vi "b2.vi"   [LabVIEW 2020]
uses:
  <instrlib>/Agilent B2900 Series/Agilent B2900 Series.lvlib
  <instrlib>/Agilent B2900 Series/Public/Data/Low Level/Fetch Measurement (Multiple Points).vi
  <instrlib>/Agilent B2900 Series/Public/Configure/Measurement/Configure Measurement (Resistance).vi
  <instrlib>/Agilent B2900 Series/Public/Data/Read Measurement Result (Single Point).vi
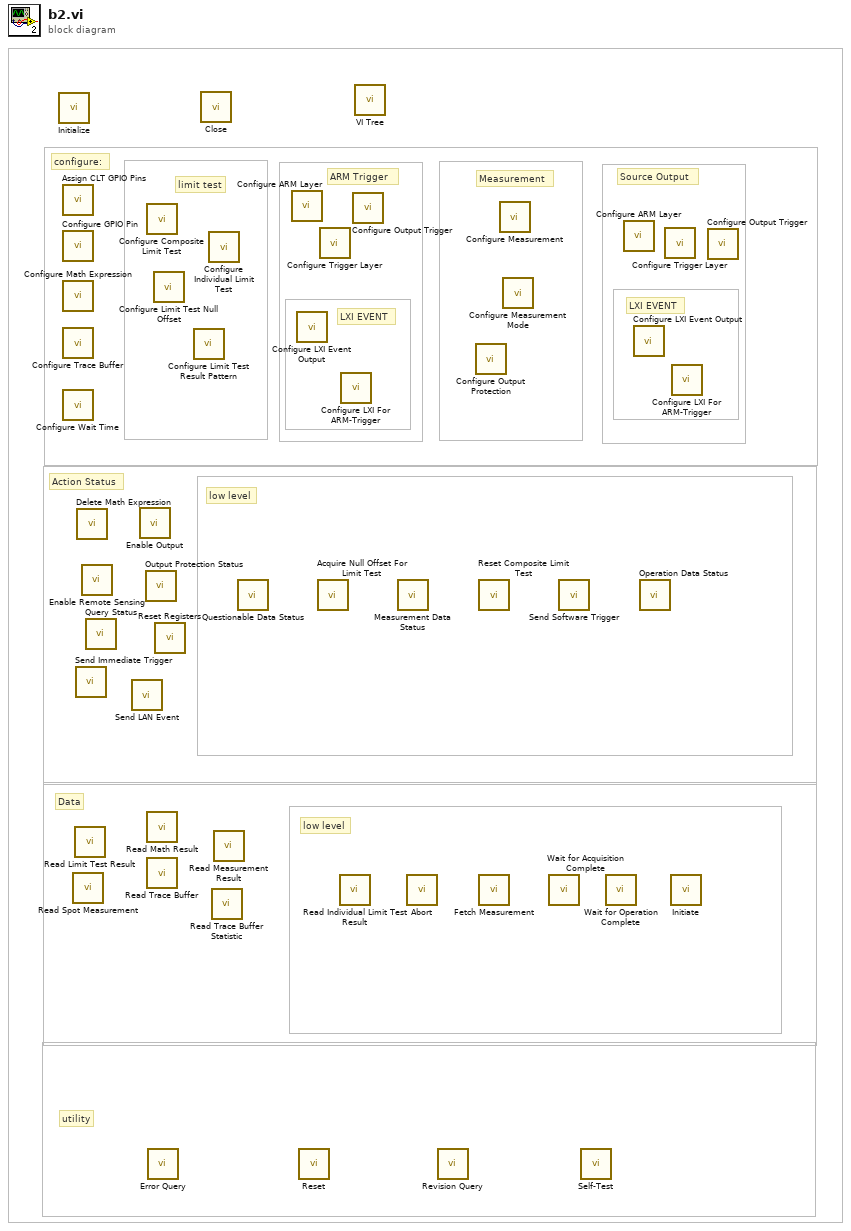
[diagram p0: block diagram]
diagram:
  # "utility"
  # "low level"
  # "low level"
  # "Data"
  # "Action Status"
  # "Source Output"
  # "Measurement"
  # "LXI EVENT"
  # "LXI EVENT"
  # "ARM Trigger"
  # "limit test"
  # "configure:"
  n1 = call <instrlib>:"Initialize.vi"() -> ()  [unwired: 10 in, 2 out]
  n2 = call <instrlib>:"Assign CLT GPIO Pins.vi"() -> ()  [unwired: 10 in, 2 out]
  n3 = call <instrlib>:"Configure GPIO Pin.vi"() -> ()  [unwired: 14 in, 2 out]
  n4 = call <instrlib>:"Configure Math Expression.vi"() -> ()  [unwired: 10 in, 2 out]
  n5 = call <instrlib>:"Configure Trace Buffer.vi"() -> ()  [unwired: 10 in, 2 out]
  n6 = call <instrlib>:"Configure Wait Time.vi"() -> ()  [unwired: 14 in, 2 out]
  n7 = call <instrlib>:"Read Spot Measurement.vi"() -> ()  [unwired: 9 in, 3 out]
  n8 = call <instrlib>:"Read Limit Test Result.vi"() -> ()  [unwired: 8 in, 4 out]
  n9 = call <instrlib>:"Send Immediate Trigger.vi"() -> ()  [unwired: 10 in, 2 out]
  n10 = call <instrlib>:"Delete Math Expression.vi"() -> ()  [unwired: 10 in, 2 out]
  n11 = call <instrlib>:"Enable Remote Sensing.vi"() -> ()  [unwired: 10 in, 2 out]
  n12 = call <instrlib>:"Query Status.vi"() -> ()  [unwired: 12 in, 4 out]
  n13 = call <instrlib>:"Send LAN Event.vi"() -> ()  [unwired: 10 in, 2 out]
  n14 = call <instrlib>:"Enable Output.vi"() -> ()  [unwired: 9 in, 3 out]
  n15 = call <instrlib>:"Output Protection Status.vi"() -> ()  [unwired: 8 in, 4 out]
  n16 = call <instrlib>:"Configure Composite Limit Test.vi"() -> ()  [unwired: 14 in, 2 out]
  n17 = call <instrlib>:"Read Math Result.vi"() -> ()  [unwired: 9 in, 3 out]
  n18 = call <instrlib>:"Read Trace Buffer.vi"() -> ()  [unwired: 9 in, 3 out]
  n19 = call <instrlib>:"Error Query.vi"() -> ()  [unwired: 8 in, 4 out]
  n20 = call <instrlib>:"Configure Limit Test Null Offset.vi"() -> ()  [unwired: 10 in, 2 out]
  n21 = call <instrlib>:"Reset Registers.vi"() -> ()  [unwired: 10 in, 2 out]
  n22 = call <instrlib>:"Configure Limit Test Result Pattern.vi"() -> ()  [unwired: 14 in, 2 out]
  n23 = call <instrlib>:"Close.vi"() -> ()  [unwired: 11 in, 1 out]
  n24 = call <instrlib>:"Configure Individual Limit Test.vi"() -> ()  [unwired: 14 in, 2 out]
  n25 = call <instrlib>:"Read Trace Buffer Statistic.vi"() -> ()  [unwired: 9 in, 3 out]
  n26 = call-poly <instrlib>:"Read Measurement Result.vi"() -> ()  [unwired: 9 in, 3 out]
  n27 = call <instrlib>:"Questionable Data Status.vi"() -> ()  [unwired: 9 in, 3 out]
  n28 = call <instrlib>:"Configure ARM Layer.vi"() -> ()  [unwired: 14 in, 2 out]
  n29 = call <instrlib>:"Configure LXI Event Output.vi"() -> ()  [unwired: 14 in, 2 out]
  n30 = call <instrlib>:"Reset.vi"() -> ()  [unwired: 10 in, 2 out]
  n31 = call <instrlib>:"Acquire Null Offset For Limit Test.vi"() -> ()  [unwired: 9 in, 3 out]
  n32 = call <instrlib>:"Configure Trigger Layer.vi"() -> ()  [unwired: 14 in, 2 out]
  n33 = call <instrlib>:"Read Individual Limit Test Result.vi"() -> ()  [unwired: 9 in, 3 out]
  n34 = call <instrlib>:"Configure LXI For ARM-Trigger.vi"() -> ()  [unwired: 14 in, 2 out]
  n35 = call <instrlib>:"Configure Output Trigger.vi"() -> ()  [unwired: 14 in, 2 out]
  n36 = call <instrlib>:"VI Tree.vi"() -> ()  [unwired: 12 in]
  n37 = call <instrlib>:"Measurement Data Status.vi"() -> ()  [unwired: 9 in, 3 out]
  n38 = call <instrlib>:"Abort.vi"() -> ()  [unwired: 10 in, 2 out]
  n39 = call <instrlib>:"Revision Query.vi"() -> ()  [unwired: 8 in, 4 out]
  n40 = call <instrlib>:"Configure Output Protection.vi"() -> ()  [unwired: 10 in, 2 out]
  n41 = call <instrlib>:"Reset Composite Limit Test.vi"() -> ()  [unwired: 10 in, 2 out]
  n42 = call-poly <instrlib>:"Fetch Measurement.vi"() -> ()  [unwired: 9 in, 3 out]
  n43 = call-poly <instrlib>:"Configure Measurement.vi"() -> ()  [unwired: 18 in, 2 out]
  n44 = call <instrlib>:"Configure Measurement Mode.vi"() -> ()  [unwired: 10 in, 2 out]
  n45 = call <instrlib>:"Wait for Acquisition Complete.vi"() -> ()  [unwired: 10 in, 2 out]
  n46 = call <instrlib>:"Send Software Trigger.vi"() -> ()  [unwired: 10 in, 2 out]
  n47 = call <instrlib>:"Self-Test.vi"() -> ()  [unwired: 8 in, 4 out]
  n48 = call <instrlib>:"Wait for Operation Complete.vi"() -> ()  [unwired: 10 in, 2 out]
  n49 = call <instrlib>:"Configure ARM Layer.vi"() -> ()  [unwired: 14 in, 2 out]
  n50 = call <instrlib>:"Configure LXI Event Output.vi"() -> ()  [unwired: 14 in, 2 out]
  n51 = call <instrlib>:"Operation Data Status.vi"() -> ()  [unwired: 9 in, 3 out]
  n52 = call <instrlib>:"Configure Trigger Layer.vi"() -> ()  [unwired: 14 in, 2 out]
  n53 = call <instrlib>:"Initiate.vi"() -> ()  [unwired: 10 in, 2 out]
  n54 = call <instrlib>:"Configure LXI For ARM-Trigger.vi"() -> ()  [unwired: 14 in, 2 out]
  n55 = call <instrlib>:"Configure Output Trigger.vi"() -> ()  [unwired: 14 in, 2 out]
